vi "LVstring2C.vi"(4 "LVString":string) -> (0 "size_out":i32, 1 "CString":u8[](array[numeric]))   [LabVIEW 2019]
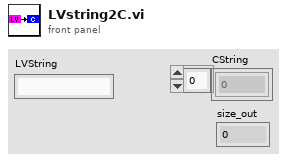
[diagram p1: front panel]
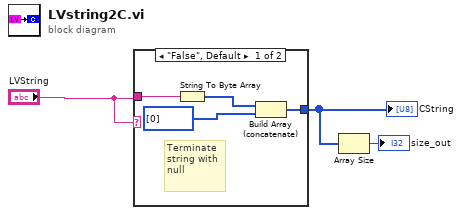
[diagram p0: block diagram]
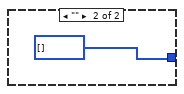
[diagram p2: hidden frame]
diagram:
  n1 = case shown="\"False\", Default" "LVString" {
    tunnel: "LVString" -> [w7 _]
    tunnel: [w4 u8[] []] -> w2
    frame "False", Default {
      # "Terminate string with null"
      n2 = String To Byte Array(string=w7) -> (unsigned byte array=w6:u8[])
      n3 = Build Array (concatenate)(w6, u8[] [0] ("array")) -> (w4:u8[])
    }
    frame "" {
    }
  }
  "CString" <- w2
  n4 = Array Size(array=w2) -> (size(s)=→"size_out":i32)
